vi "Periodic Tasks.vi"(8 "error in":errorcluster) -> ()   [LabVIEW 2014]
doc: "This VI runs in parallel to other tasks. It can contain as many user-defined periodic loops as you need. These can carry out PID or other sorts of timed response."
uses:
  <vilib>/Rock Robotics/WPI/Solenoid/WPI_SolenoidValue.ctl
  <vilib>/Rock Robotics/WPI/Joystick/WPI_JoystickGetSetRefNum.vi
  <vilib>/Rock Robotics/WPI/RobotDrive/WPI_RobotDriveGetSetRefNum.vi
  Robot Global Data.vi
  <vilib>/Rock Robotics/Network Tables/SD Write String.vi
  <vilib>/Rock Robotics/WPI/Solenoid/WPI_SolenoidSetEnum.vi
panel:
  out "Photoeye":bool
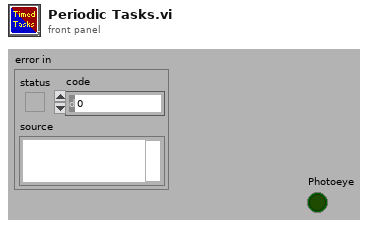
[diagram p1: front panel]
types:
  T1 = typedef "WPI_SolenoidValue.ctl" = enum16{"Off", "On", "Forward", "Reverse"}
  T2 = typedef "WPI_JoystickDevRef.ctl" = cluster{"Device":T3}
  T3 = typedef "WPI_JoystickDeviceEnum.ctl" = enum16{"USB 0", "USB 1", "USB 2", "USB 3", "USB 4", "USB 5"}
  T4 = typedef "WPI_RobotDriveDevRef.ctl" = cluster{"DevStatus":errorcluster, "Motors[]":T5[], "Square Inputs":bool, "Max Output":dbl}
  T5 = typedef "WPI_MotorControlDeviceRef.ctl" = cluster{"DeviceStatus":errorcluster, "Type":T6, "PWM":cluster{"Controller":T7, "PWM Channel":T8, "DeadBand":T9}, "CAN":cluster{"Device Number":u8, "Control Mode":T10, "Semaphore":T11, "Max Vout":dbl, "TalonSRX Control Mode":T12}, "Invert":bool, "TransformRef":T13, "InvTransformRef":T13}
  T6 = typedef "WPI_MotorControlType.ctl" = enum16{"PWM", "CAN", "CANTalonSRX"}
  T7 = typedef "FPGA_TypedefDigitalModule.ctl" = enum16{"Controller 1"}
  T8 = typedef "FPGA_DIOPWMChannel.ctl" = enum8{"PWM 0", "PWM 1", "PWM 2", "PWM 3", "PWM 4", "PWM 5", "PWM 6", "PWM 7", "PWM 8", "PWM 9", "PWM MXP 0", "PWM MXP 1", "PWM MXP 2", "PWM MXP 3", "PWM MXP 4", "PWM MXP 5", "PWM MXP 6", "PWM MXP 7", "PWM MXP 8", "PWM MXP 9", "Invalid"}
  T9 = typedef "WPI_PWMDeadband.ctl" = cluster{"Name":string, "maxPositivePwm":i32, "minPositivePwm":i32, "centerPwm":i32, "maxNegativePwm":i32, "minNegativePwm":i32, "angularRange":u16}
  T10 = typedef "WPI_CANJaguar_ControlMode.ctl" = enum8{"Percent VBus", "Current", "Speed", "Position", "Voltage"}
  T11 = typedef "Semaphore RefNum" = refnum<k1>
  T12 = typedef "WPI_CANTalonSRX_APIControlMode.ctl" = enum8{"Percent VBus", "Speed", "Position", "Slave", "Unchanged / Invalid"}
  T13 = typedef "WPI_PWMTransform_ConPane.ctl" = refnum<vi>
  T14 = cluster{"JoystickDevRef":T2, "RobotDriveDevRef":T4}
  T15 = typedef "WPI_DigitalInputDevRef.ctl" = cluster{"DevStatus":errorcluster, "DIO Channel":T16, "Controller":T7}
  T16 = typedef "FPGA_DIOChannel.ctl" = enum8{"DIO 0", "DIO 1", "DIO 2", "DIO 3", "DIO 4", "DIO 5", "DIO 6", "DIO 7", "DIO 8", "DIO 9", "DIO MXP 0", "DIO MXP 1", "DIO MXP 2", "DIO MXP 3", "DIO MXP 4", "DIO MXP 5", "DIO MXP 6", "DIO MXP 7", "DIO MXP 8", "DIO MXP 9", "DIO MXP 10", "DIO MXP 11", "DIO MXP 12", "DIO MXP 13", "DIO MXP 14", "DIO MXP 15", "Invalid"}
  T17 = typedef "WPI_SolenoidDevRef.ctl" = cluster{"DevStatus":errorcluster, "Pneumatics Control Module":u8, "Forward Solenoid Channel":T18, "Reverse Solenoid Channel":T18}
  T18 = typedef "WPI_SolenoidChannel.ctl" = enum8{"Solenoid 0", "Solenoid 1", "Solenoid 2", "Solenoid 3", "Solenoid 4", "Solenoid 5", "Solenoid 6", "Solenoid 7", "Invalid"}
  T19 = typedef "WPI_ServoDeviceRef.ctl" = cluster{"DeviceStatus":errorcluster, "Controller":T7, "PWM Channel":T8, "DeadBand":T9}
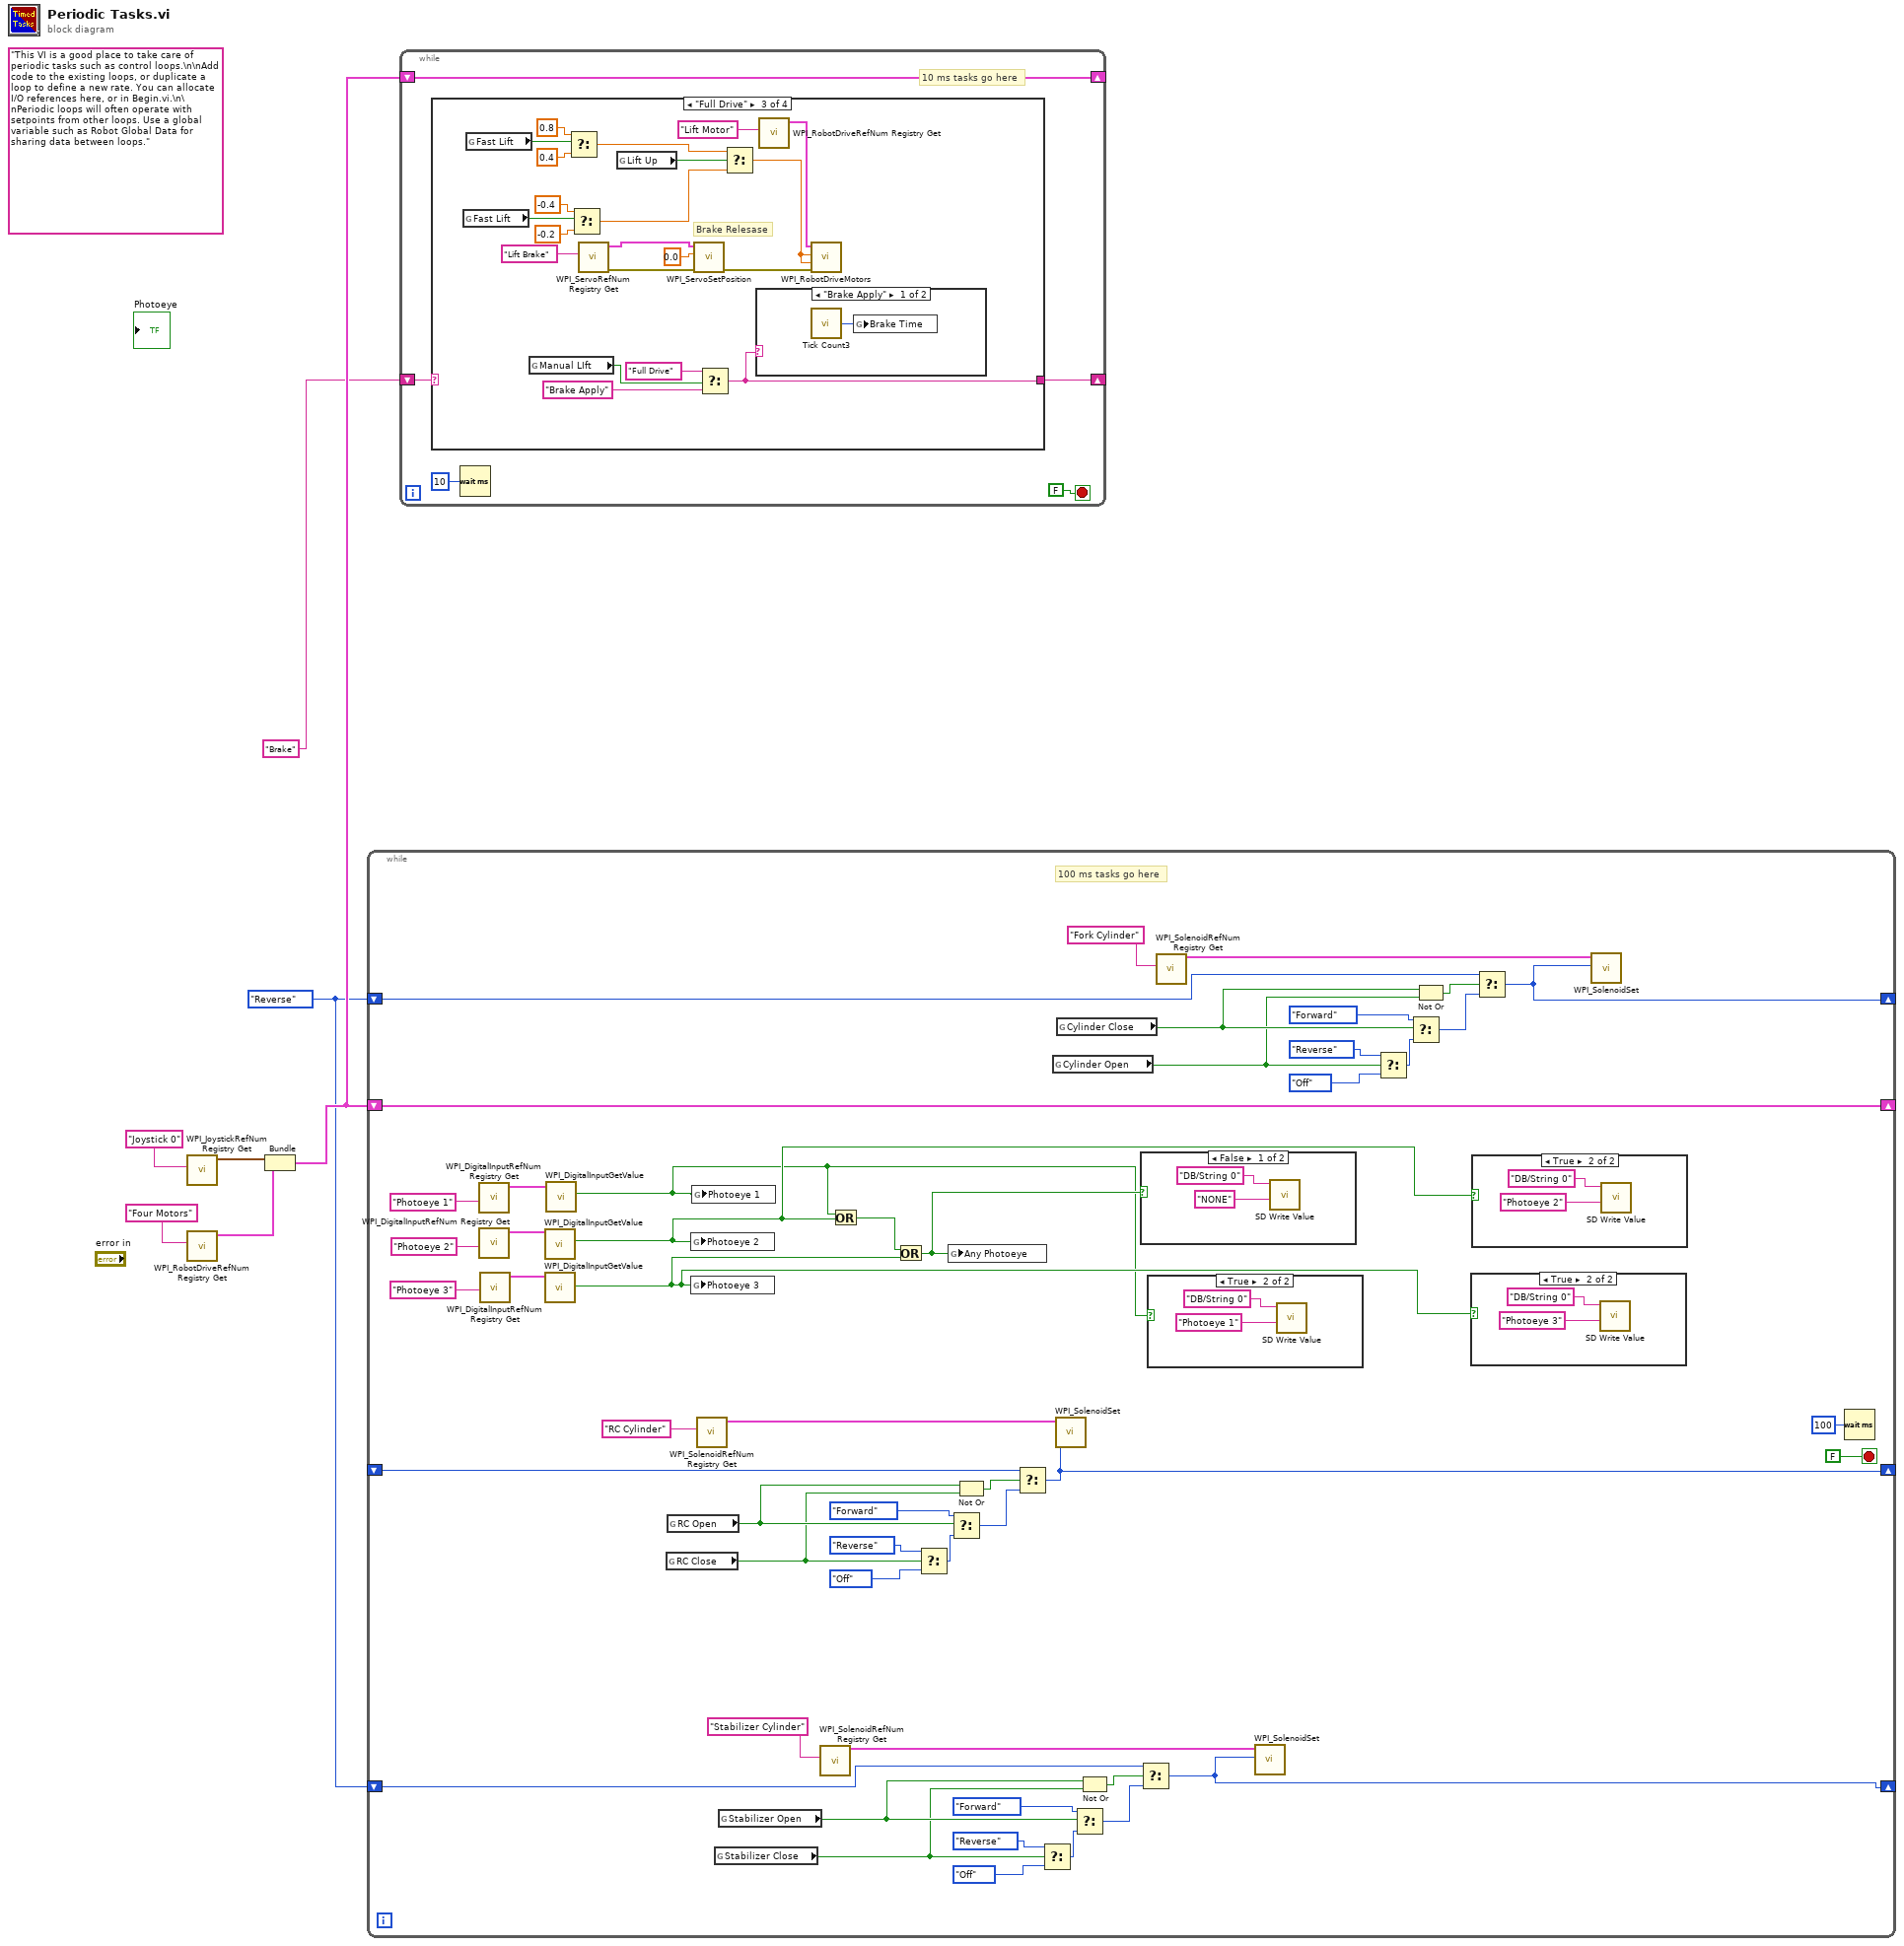
[diagram p0: block diagram]
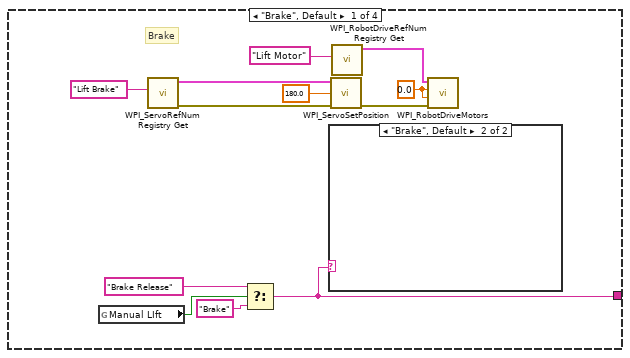
[diagram p6: hidden frame]
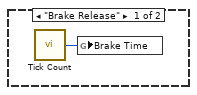
[diagram p7: hidden frame]
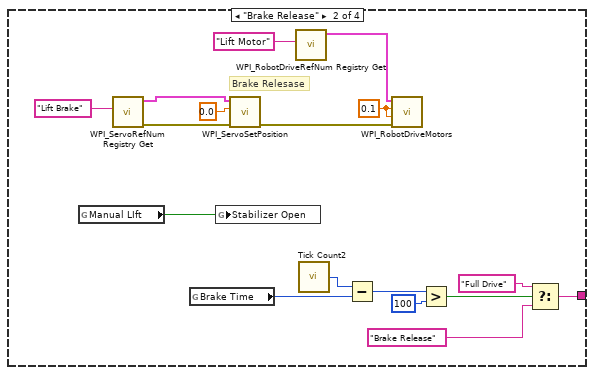
[diagram p8: hidden frame]
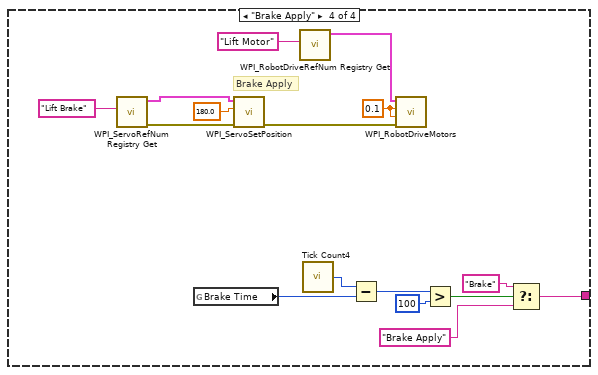
[diagram p10: hidden frame]
diagram:
  w1 = WPI_SolenoidValue."Reverse" ("Value")
  (unwired) "This VI is a good place to take care of periodic tasks such as control loops.\n\nAdd code to the existing loops, or duplicate a loop to define a new rate. You can allocate I/O references here, or in Begin.vi.\n\nPeriodic loops will often operate with setpoints from other loops. Use a global variable such as Robot Global Data for sharing data between loops."
  n1 = call <vilib>:"WPI_JoystickRefNum Registry Get.vi"("refnum name"="Joystick 0") -> ("JoystickDevRef"=w5:T2)  [unwired: 1 in, 9 out]
  n2 = call <vilib>:"WPI_RobotDriveRefNum Registry Get.vi"("refnum name"="Four Motors") -> ("RobotDriveDevRef"=w4:T4)  [unwired: 1 in, 9 out]
  n3 = Bundle("JoystickDevRef"=w5, "RobotDriveDevRef"=w4) -> (w3:T14)  [unwired: 1 out]
  n4 = while {
    shift-right: [w55] -> _
    shift-left: w3 -> [w55]
    shift-right: [w47] -> _
    shift-left: w1 -> [w46]
    shift-right: [w23] -> _
    shift-left: _ -> [w22]
    shift-right: [w9] -> _
    shift-left: w1 -> [w8]
    stop <- FALSE stop-if-true
    # "100 ms tasks go here"
    n5 = call <vilib>:"WPI_DigitalInputRefNum Registry Get.vi"("refnum name"="Photoeye 1") -> ("DigitalInputDevRef"=w41:T15)  [unwired: 9 in, 1 out]
    n6 = call <vilib>:"WPI_DigitalInputRefNum Registry Get.vi"("refnum name"="Photoeye 2") -> ("DigitalInputDevRef"=w39:T15)  [unwired: 9 in, 1 out]
    n7 = call <vilib>:"WPI_DigitalInputRefNum Registry Get.vi"("refnum name"="Photoeye 3") -> ("DigitalInputDevRef"=w38:T15)  [unwired: 9 in, 1 out]
    n8 = call <vilib>:"WPI_DigitalInputGetValue.vi"("DigitalInputDevRef"=w39) -> ("Value"=w33:bool)  [unwired: 8 in, 2 out]
    n9 = call <vilib>:"WPI_DigitalInputGetValue.vi"("DigitalInputDevRef"=w38) -> ("Value"=w34:bool)  [unwired: 8 in, 2 out]
    n10 = call <vilib>:"WPI_DigitalInputGetValue.vi"("DigitalInputDevRef"=w41) -> ("Value"=w32:bool)  [unwired: 8 in, 2 out]
    n11 = global read "Robot Global Data.vi" "RC Close"() -> (w20:bool)
    n12 = global read "Robot Global Data.vi" "RC Open"() -> (w21:bool)
    n13 = global write "Robot Global Data.vi" "Photoeye 2"(w33) -> ()
    n14 = global write "Robot Global Data.vi" "Photoeye 3"(w34) -> ()
    n15 = global write "Robot Global Data.vi" "Photoeye 1"(w32) -> ()
    n16 = call <vilib>:"WPI_SolenoidRefNum Registry Get.vi"("refnum name"="RC Cylinder") -> ("SolenoidDevRef"=w26:T17)  [unwired: 9 in, 1 out]
    n17 = global read "Robot Global Data.vi" "Stabilizer Close"() -> (w10:bool)
    n18 = global read "Robot Global Data.vi" "Stabilizer Open"() -> (w11:bool)
    n19 = call <vilib>:"WPI_SolenoidRefNum Registry Get.vi"("refnum name"="Stabilizer Cylinder") -> ("SolenoidDevRef"=w14:T17)  [unwired: 9 in, 1 out]
    n20 = Or(x=w32, y=w33) -> (x .or. y?=w36:bool)
    n21 = Or(x=w36, y=w34) -> (x .or. y?=w35:bool)
    n22 = Select(t=WPI_SolenoidValue."Reverse" ("Value"), s=w20, f=WPI_SolenoidValue."Off" ("Value")) -> (s? t:f=w28:T1)
    n23 = global write "Robot Global Data.vi" "Any Photoeye"(w35) -> ()
    n24 = Select(t=WPI_SolenoidValue."Forward" ("Value"), s=w21, f=w28) -> (s? t:f=w25:T1)
    n25 = Not Or(1:w20, 2:w21) -> (0:w24:bool)
    n26 = Select(t=w22, s=w24, f=w25) -> (s? t:f=w23:T1)
    n27 = Select(t=WPI_SolenoidValue."Reverse" ("Value"), s=w10, f=WPI_SolenoidValue."Off" ("Value")) -> (s? t:f=w16:T1)
    n28 = global read "Robot Global Data.vi" "Cylinder Open"() -> (w43:bool)
    n29 = call-poly <vilib>:"WPI_SolenoidSet.vi"("Value"=w23, "SolenoidDevRef"=w26) -> ()  [unwired: 1 in, 9 out]
    n30 = global read "Robot Global Data.vi" "Cylinder Close"() -> (w44:bool)
    n31 = Select(t=WPI_SolenoidValue."Forward" ("Value"), s=w11, f=w16) -> (s? t:f=w13:T1)
    n32 = Not Or(1:w10, 2:w11) -> (0:w12:bool)
    n33 = case shown="False" w35 {
      frame False {
        n34 = call-poly <vilib>:"SD Write Value.vi"("String"="NONE", "Name"="DB/String 0") -> ()  [unwired: 8 in, 2 out]
      }
      frame True {
      }
    }
    n35 = Select(t=w8, s=w12, f=w13) -> (s? t:f=w9:T1)
    n36 = case shown="True" w32 {
      frame False {
      }
      frame True {
        n37 = call-poly <vilib>:"SD Write Value.vi"("String"="Photoeye 1", "Name"="DB/String 0") -> ()  [unwired: 8 in, 2 out]
      }
    }
    n38 = call <vilib>:"WPI_SolenoidRefNum Registry Get.vi"("refnum name"="Fork Cylinder") -> ("SolenoidDevRef"=w49:T17)  [unwired: 9 in, 1 out]
    n39 = call-poly <vilib>:"WPI_SolenoidSet.vi"("Value"=w9, "SolenoidDevRef"=w14) -> ()  [unwired: 1 in, 9 out]
    n40 = Select(t=WPI_SolenoidValue."Reverse" ("Value"), s=w43, f=WPI_SolenoidValue."Off" ("Value")) -> (s? t:f=w51:T1)
    n41 = Select(t=WPI_SolenoidValue."Forward" ("Value"), s=w44, f=w51) -> (s? t:f=w48:T1)
    n42 = Not Or(1:w43, 2:w44) -> (0:w45:bool)
    n43 = case shown="True" w34 {
      frame False {
      }
      frame True {
        n44 = call-poly <vilib>:"SD Write Value.vi"("String"="Photoeye 3", "Name"="DB/String 0") -> ()  [unwired: 8 in, 2 out]
      }
    }
    n45 = case shown="True" w33 {
      frame False {
      }
      frame True {
        n46 = call-poly <vilib>:"SD Write Value.vi"("String"="Photoeye 2", "Name"="DB/String 0") -> ()  [unwired: 8 in, 2 out]
      }
    }
    n47 = Select(t=w46, s=w45, f=w48) -> (s? t:f=w47:T1)
    n48 = call-poly <vilib>:"WPI_SolenoidSet.vi"("Value"=w47, "SolenoidDevRef"=w49) -> ()  [unwired: 1 in, 9 out]
    n49 = Wait (ms)(milliseconds to wait=u32 100) -> ()  [unwired: 1 out]
  }
  n50 = while {
    shift-right: [w68] -> _
    shift-left: w3 -> [w68]
    shift-right: [w67] -> _
    shift-left: "Brake" -> [w66]
    stop <- FALSE stop-if-true
    # "10 ms tasks go here"
    n51 = case shown="\"Full Drive\"" w66 {
      tunnel: [w71 w85 w109 w123] -> w67
      frame "Brake", Default {
        w77 = 0.0 ("LeftSpeed")
        # "Brake"
        n52 = global read "Robot Global Data.vi" "Manual LIft"() -> (w74:bool)
        n53 = call <vilib>:"WPI_ServoRefNum Registry Get.vi"("refnum name"="Lift Brake") -> ("error out"=w75:errorcluster, "ServoDeviceRef"=w80:T19)  [unwired: 9 in]
        n54 = Select(t="Brake Release", s=w74, f="Brake") -> (s? t:f=w71:string)
        n55 = case shown="\"Brake\", Default" w71 {
          frame "Brake Release" {
            n56 = call "Tick Count"() -> ("Tick Count(mSec)"=w83:u32)
            n57 = global write "Robot Global Data.vi" "Brake Time"(w83) -> ()
          }
          frame "Brake", Default {
          }
        }
        n58 = call <vilib>:"WPI_ServoSetPosition.vi"("error in (no error)"=w75, "Position"=180.0, "ServoDeviceRef"=w80) -> ("error out"=w76:errorcluster)  [unwired: 7 in, 1 out]
        n59 = call <vilib>:"WPI_RobotDriveRefNum Registry Get.vi"("refnum name"="Lift Motor") -> ("RobotDriveDevRef"=w78:T4)  [unwired: 9 in, 1 out]
        n60 = call <vilib>:"WPI_RobotDriveMotors.vi"("error in (no error)"=w76, "RightSpeed"=w77, "LeftSpeed"=w77, "RobotDriveDevRef"=w78) -> ()  [unwired: 5 in, 3 out]
      }
      frame "Brake Release" {
        w93 = 0.1 ("RightSpeed")
        # "Brake Relesase"
        n61 = global read "Robot Global Data.vi" "Manual LIft"() -> (w84:bool)
        n62 = call <vilib>:"WPI_ServoRefNum Registry Get.vi"("refnum name"="Lift Brake") -> ("error out"=w95:errorcluster, "ServoDeviceRef"=w98:T19)  [unwired: 9 in]
        n63 = global read "Robot Global Data.vi" "Brake Time"() -> (w86:u32)
        n64 = global write "Robot Global Data.vi" "Stabilizer Open"(w84) -> ()
        n65 = call <vilib>:"WPI_ServoSetPosition.vi"("error in (no error)"=w95, "Position"=0.0, "ServoDeviceRef"=w98) -> ("error out"=w94:errorcluster)  [unwired: 7 in, 1 out]
        n66 = call <vilib>:"WPI_RobotDriveRefNum Registry Get.vi"("refnum name"="Lift Motor") -> ("RobotDriveDevRef"=w96:T4)  [unwired: 9 in, 1 out]
        n67 = call "Tick Count2"() -> ("Tick Count(mSec)"=w87:u32)
        n68 = Subtract(x=w87, y=w86) -> (x-y=w90:u32)
        n69 = call <vilib>:"WPI_RobotDriveMotors.vi"("error in (no error)"=w94, "RightSpeed"=w93, "LeftSpeed"=w93, "RobotDriveDevRef"=w96) -> ()  [unwired: 5 in, 3 out]
        n70 = Greater?(x=w90, y=u32 100) -> (0:w91:bool)
        n71 = Select(t="Full Drive", s=w91, f="Brake Release") -> (s? t:f=w85:string)
      }
      frame "Full Drive" {
        # "Brake Relesase"
        n72 = global read "Robot Global Data.vi" "Fast Lift"() -> (w108:bool)
        n73 = global read "Robot Global Data.vi" "Fast Lift"() -> (w104:bool)
        n74 = global read "Robot Global Data.vi" "Manual LIft"() -> (w112:bool)
        n75 = Select(t=0.8 ("f"), s=w104, f=0.4) -> (s? t:f=w101:dbl)
        n76 = Select(t=-0.4 ("f"), s=w108, f=-0.2) -> (s? t:f=w105:dbl)
        n77 = call <vilib>:"WPI_ServoRefNum Registry Get.vi"("refnum name"="Lift Brake") -> ("error out"=w116:errorcluster, "ServoDeviceRef"=w119:T19)  [unwired: 9 in]
        n78 = global read "Robot Global Data.vi" "Lift Up"() -> (w113:bool)
        n79 = call <vilib>:"WPI_ServoSetPosition.vi"("error in (no error)"=w116, "Position"=0.0, "ServoDeviceRef"=w119) -> ("error out"=w115:errorcluster)  [unwired: 7 in, 1 out]
        n80 = Select(t="Full Drive", s=w112, f="Brake Apply") -> (s? t:f=w109:string)
        n81 = Select(t=w101, s=w113, f=w105) -> (s? t:f=w114:dbl)
        n82 = case shown="\"Brake Apply\"" w109 {
          frame "Brake Apply" {
            n83 = call "Tick Count3"() -> ("Tick Count(mSec)"=w122:u32)
            n84 = global write "Robot Global Data.vi" "Brake Time"(w122) -> ()
          }
          frame "Full Drive", Default {
          }
        }
        n85 = call <vilib>:"WPI_RobotDriveRefNum Registry Get.vi"("refnum name"="Lift Motor") -> ("RobotDriveDevRef"=w117:T4)  [unwired: 9 in, 1 out]
        n86 = call <vilib>:"WPI_RobotDriveMotors.vi"("error in (no error)"=w115, "RightSpeed"=w114, "LeftSpeed"=w114, "RobotDriveDevRef"=w117) -> ()  [unwired: 5 in, 3 out]
      }
      frame "Brake Apply" {
        w138 = 0.1 ("RightSpeed")
        # "Brake Apply"
        n87 = call <vilib>:"WPI_ServoRefNum Registry Get.vi"("refnum name"="Lift Brake") -> ("error out"=w136:errorcluster, "ServoDeviceRef"=w133:T19)  [unwired: 9 in]
        n88 = global read "Robot Global Data.vi" "Brake Time"() -> (w125:u32)
        n89 = call <vilib>:"WPI_ServoSetPosition.vi"("error in (no error)"=w136, "Position"=180.0, "ServoDeviceRef"=w133) -> ("error out"=w137:errorcluster)  [unwired: 7 in, 1 out]
        n90 = call <vilib>:"WPI_RobotDriveRefNum Registry Get.vi"("refnum name"="Lift Motor") -> ("RobotDriveDevRef"=w135:T4)  [unwired: 9 in, 1 out]
        n91 = call "Tick Count4"() -> ("Tick Count(mSec)"=w126:u32)
        n92 = Subtract(x=w126, y=w125) -> (x-y=w124:u32)
        n93 = call <vilib>:"WPI_RobotDriveMotors.vi"("error in (no error)"=w137, "RightSpeed"=w138, "LeftSpeed"=w138, "RobotDriveDevRef"=w135) -> ()  [unwired: 5 in, 3 out]
        n94 = Greater?(x=w124, y=u32 100) -> (0:w127:bool)
        n95 = Select(t="Brake", s=w127, f="Brake Apply") -> (s? t:f=w123:string)
      }
    }
    n96 = Wait (ms)(milliseconds to wait=u32 10) -> ()  [unwired: 1 out]
  }
